vi "mainpanel.vi"() -> ()   [LabVIEW 2020]
panel:
  out "布尔":bool
  in  "混响吸声测量":bool
  in  "基本测量":bool
  in  "退出":bool
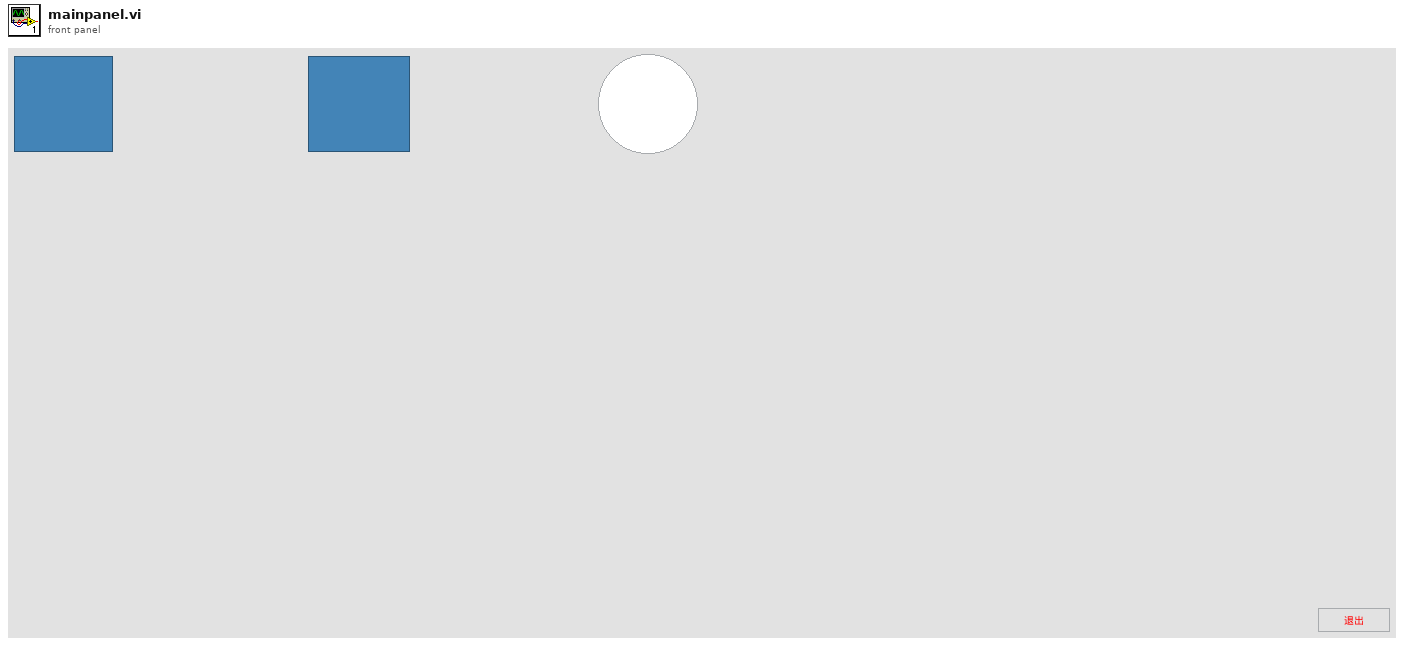
[diagram p1: front panel]
types:
  T1 = enum32{"Invalid", "Standard", "Closed", "Hidden", "Minimized", "Maximized"}
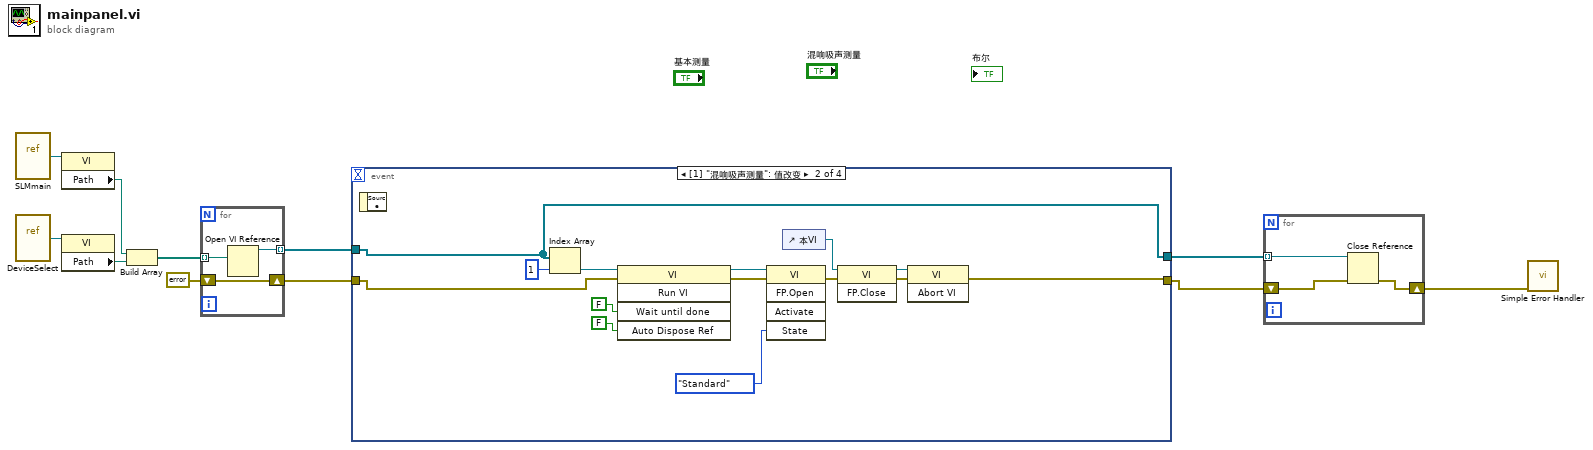
[diagram p0: block diagram]
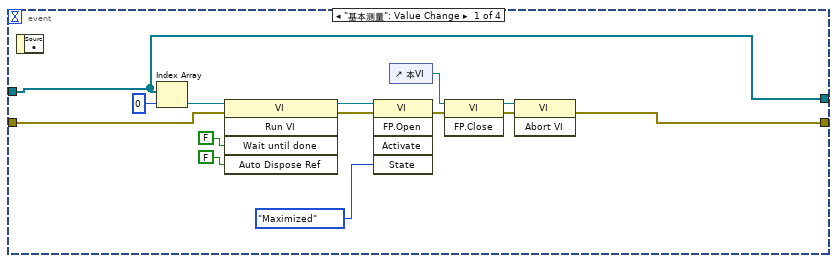
[diagram p2: hidden frame]
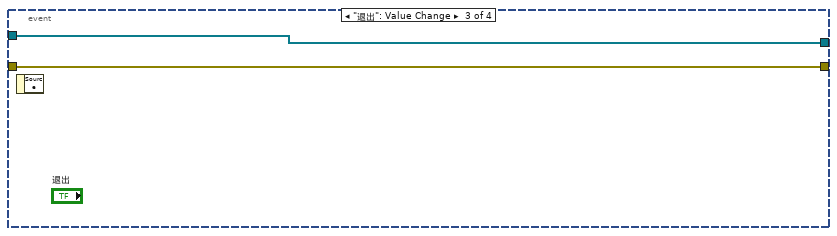
[diagram p3: hidden frame]
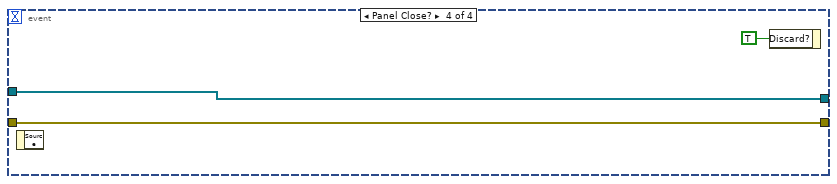
[diagram p4: hidden frame]
diagram:
  n1 = vi-ref "SLMmain.vi"() -> (w7:refnum<vi>)
  n2 = vi-ref "DeviceSelect.vi"() -> (w6:refnum<vi>)
  n3 = property class="VI"(reference=w7) -> ("Path"=w5:path)  [unwired: 1 in, 2 out]
  n4 = property class="VI"(reference=w6) -> ("Path"=w4:path)  [unwired: 1 in, 2 out]
  n5 = Build Array(w5, w4) -> (w11:path[])
  n6 = for {
    tunnel: w11 -> [w12] mode=indexing
    shift-right: [w13] -> w8
    shift-left: errorcluster {"status"=FALSE, "code"=0, "source"=""} ("错误输入（无错误）") -> [w13]
    tunnel: [w14] -> w9 mode=indexing
    n7 = Open VI Reference(vi path=w12) -> (vi reference=w14:refnum<vi>)  [unwired: 5 in, 1 out]
  }
  n8 = event shown="[1] \"混响吸声测量\": 值改变" {
    selector: _ -> [_ _ _ _]
    dyn-events: _ -> [_ _ _ _]
    timeout: _ -> [_ _ _ _]
    tunnel: w9 -> [w16 w29 w43 w46]
    tunnel: w8 -> [w19 w31 w44 w45]
    tunnel: [w15 w30 w44 w45] -> w1
    tunnel: [w16 w29 w43 w46] -> w2
    event "基本测量": Value Change {
      n9 = event-data() -> ()  [unwired: 1 in, 1 out]
      n10 = Index Array(array=w16, index=0 ("索引")) -> (element=w26:refnum<vi>)
      n11 = invoke class="VI" method="Run VI"(reference=w26, error in=w19, "Wait until done"=FALSE ("结束前等待"), "Auto Dispose Ref"=FALSE ("自动销毁引用")) -> (reference out=w21:refnum<vi>, error out=w20:errorcluster)  [unwired: 1 in, 3 out]
      n12 = invoke class="VI" method="FP.Open"(reference=w21, error in=w20, "State"=T1."Maximized" ("状态")) -> (error out=w25:errorcluster)  [unwired: 2 in, 4 out]
      n13 = control-ref of="本VI"() -> (w17:refnum<vi>)
      n14 = invoke class="VI" method="FP.Close"(reference=w17, error in=w25) -> (reference out=w24:refnum<vi>, error out=w23:errorcluster)  [unwired: 1 in, 1 out]
      n15 = invoke class="VI" method="Abort VI"(reference=w24, error in=w23) -> (error out=w15:errorcluster)  [unwired: 1 in, 2 out]
    }
    event "混响吸声测量": Value Change {
      n16 = event-data() -> ()  [unwired: 1 in, 1 out]
      n17 = Index Array(array=w29, index=1 ("索引")) -> (element=w40:refnum<vi>)
      n18 = invoke class="VI" method="Run VI"(reference=w40, error in=w31, "Wait until done"=FALSE ("结束前等待"), "Auto Dispose Ref"=FALSE ("自动销毁引用")) -> (reference out=w35:refnum<vi>, error out=w34:errorcluster)  [unwired: 1 in, 3 out]
      n19 = invoke class="VI" method="FP.Open"(reference=w35, error in=w34, "State"=T1."Standard" ("状态")) -> (error out=w39:errorcluster)  [unwired: 2 in, 4 out]
      n20 = control-ref of="本VI"() -> (w32:refnum<vi>)
      n21 = invoke class="VI" method="FP.Close"(reference=w32, error in=w39) -> (reference out=w38:refnum<vi>, error out=w37:errorcluster)  [unwired: 1 in, 1 out]
      n22 = invoke class="VI" method="Abort VI"(reference=w38, error in=w37) -> (error out=w30:errorcluster)  [unwired: 1 in, 2 out]
    }
    event "退出": Value Change {
      n23 = event-data() -> ()  [unwired: 1 in, 1 out]
    }
    event Panel Close? {
      n24 = event-data() -> ()  [unwired: 1 in, 1 out]
      n25 = event-data("Discard?"=TRUE ("放弃？")) -> ()  [unwired: 1 in, 1 out]
    }
  }
  n26 = for {
    shift-right: [w50] -> w3
    shift-left: w1 -> [w49]
    tunnel: w2 -> [w48] mode=indexing
    n27 = Close Reference(reference=w48, error in (no error)=w49) -> (error out=w50:errorcluster)
  }
  n28 = call <vilib>:"Simple Error Handler.vi"("error in (no error)"=w3) -> ()  [unwired: 4 in, 5 out]
